vi "LoadHospitalWrapper.vi"(8 "error in (no error)":errorcluster, 11 "PatientDatePath":path) -> (0 "error out":errorcluster, 1 "Address":string, 2 "Department":string, 3 "Name":string)   [LabVIEW 2013, in "main.lvlib"]
uses:
  main.lvlib
  <userlib>/_OpenG.lib/file/file.llb/File Exists - Scalar__ogtk.vi
  <vilib>/Utility/file.llb/Read From Spreadsheet File (string).vi
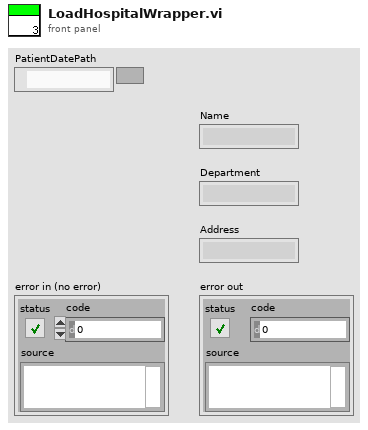
[diagram p1: front panel]
types:
  T1 = cluster{"name":string, "department":string, "address":string}
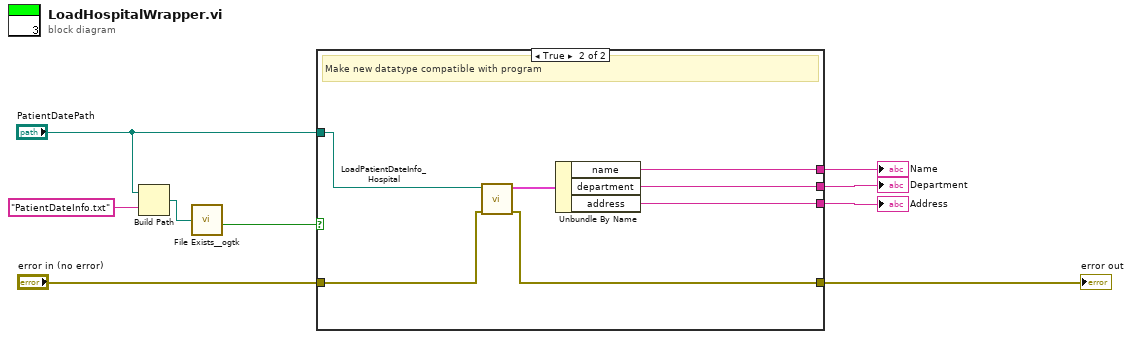
[diagram p0: block diagram]
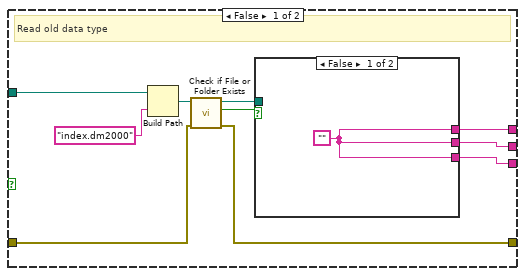
[diagram p2: hidden frame]
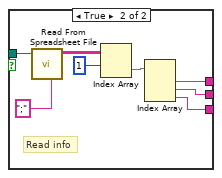
[diagram p3: hidden frame]
diagram:
  n1 = Build Path(base path="PatientDatePath", name or relative path="PatientDateInfo.txt") -> (appended path=w2:path)
  n2 = call-poly <userlib>:"File Exists__ogtk.vi"("file path"=w2) -> ("exists"=w1:bool)  [unwired: 6 in, 1 out]
  n3 = case shown="True" w1 {
    tunnel: [w19 w34] -> w9
    tunnel: "error in (no error)" -> [w18 w35]
    tunnel: [w17 w30] -> w7
    tunnel: [w16 w31] -> w6
    tunnel: [w15 w32] -> w5
    tunnel: "PatientDatePath" -> [w10 w29]
    frame False {
      # "Read old data type"
      n4 = Build Path(base path=w10, name or relative path="index.dm2000") -> (appended path=w12:path)
      n5 = call <vilib>:"Check if File or Folder Exists.vi"("error in (no error)"=w18, "path"=w12) -> ("error out"=w19:errorcluster, "file or folder exists?"=w14:bool, "dup path"=w13:path)  [unwired: 7 in]
      n6 = case shown="False" w14 {
        tunnel: w13 -> [_ w28]
        tunnel: [w20 w23] -> w15
        tunnel: [w20 w22] -> w16
        tunnel: [w20 w21] -> w17
        frame False {
          w20 = ""
        }
        frame True {
          # "Read info"
          n7 = call-poly <vilib>:"Read From Spreadsheet File.vi"("delimiter (\\t)"=";" ("delimiter (\\t)"), "file path (dialog if empty)"=w28) -> ("all rows"=w26:string[][])  [unwired: 5 in, 4 out]
          n8 = Index Array(array=w26, index (row)=1) -> (element=w24:string[])  [unwired: 1 in]
          n9 = Index Array(array=w24) -> (element #1=w23:string, element #2=w22:string, element #3=w21:string)  [unwired: 3 in]
        }
      }
    }
    frame True {
      # "Make new datatype compatible with program"
      n10 = call "LoadPatientDateInfo_Hospital.vi"("error in (no error)"=w35, "DataPatientDatePath"=w29) -> ("error out"=w34:errorcluster, "hospital"=w33:T1)  [unwired: 8 in]
      n11 = Unbundle By Name(w33) -> ("name"=w32:string, "department"=w31:string, "address"=w30:string)
    }
  }
  "error out" <- w9
  "Address" <- w7
  "Department" <- w6
  "Name" <- w5
